vi "Define Mask.vi"(8 "error in (no error)":errorcluster, 11 "FPGA Image":T3(plugin-control)=refnum) -> (0 "error out":errorcluster)   [LabVIEW 2013]
doc: "GUI for selecting a part type and starting a batch process\nPart types list is passed in from caller.\nReturns when Start or Cancel is pressed."
uses:
  Sectors/Number of Wing Sector.ctl
  Mask ROI FG Enum.ctl
  Mask ROI Cluster.ctl
  Common/File IO/INI/Read write mode.ctl
  Message Passing/MsgQ Loops enum.ctl
  System Status/Status FG Enum.ctl
  Common/State Machines/State Machine Lib.lvlib
  Common/GUI/GUI.lvlib
  <vilib>/vision/NI_Vision_Development_Module.lvlib
  Image Processing.lvlib
  Message Passing/Main MsgQ.lvlib
panel:
  in  "Calculate BG":bool
  in  "Load Current Mask":bool
  out "Right ROI":T1 {"Contours"."Type" items=["No Selection", "Point", "Line", "Rectangle", "Oval", "Polygon", "Freehand Region", "Annulus", "Unused2", "Unused3", "Broken Line", "Freehand Line", "Rotated Rectangle"]}
  out "Left ROI":T1 {"Contours"."Type" items=["No Selection", "Point", "Line", "Rectangle", "Oval", "Polygon", "Freehand Region", "Annulus", "Unused2", "Unused3", "Broken Line", "Freehand Line", "Rotated Rectangle"]}
  out "[Avg BG]":dbl[](array[numeric])
  in  "NumWingSectors":T2=1 items=["1"=1, "2"=2, "4"=4, "8"=8, "16"=16]
  out "State":string
  in  "Exit":bool
  in  "Save Mask":bool
  out "combo mask":T3(plugin-control)
  out "right mask":T3(plugin-control)
  out "right masked image":T3(plugin-control)
  out "right annulus":T4={"Center X"=929, "Center Y"=663, "Inner Radius"=200, "Outer Radius"=405, "Start Angle"=90.0, "End Angle"=180.0} {"End Angle" format="%.2f"; "Start Angle" format="%.2f"; "Center X" scale=0.0..1024.0}
  out "left mask":T3(plugin-control)
  out "left masked image":T3(plugin-control)
  out "left annulus":T4={"Center X"=929, "Center Y"=663, "Inner Radius"=200, "Outer Radius"=405, "Start Angle"=90.0, "End Angle"=180.0} {"End Angle" format="%.2f"; "Start Angle" format="%.2f"; "Center X" scale=0.0..1024.0}
  in  "Accept Threshold":bool
  out "Processed Image":T3(plugin-control)
  in  "Threshold Range":cluster{"Lower value":dbl, "Upper value":dbl}={"Lower value"=106.82432432432432, "Upper value"=255.0} {"Upper value" min=0.0 max=255.0 scale=0.0..255.0; "Lower value" min=0.0 max=255.0 scale=0.0..255.0}
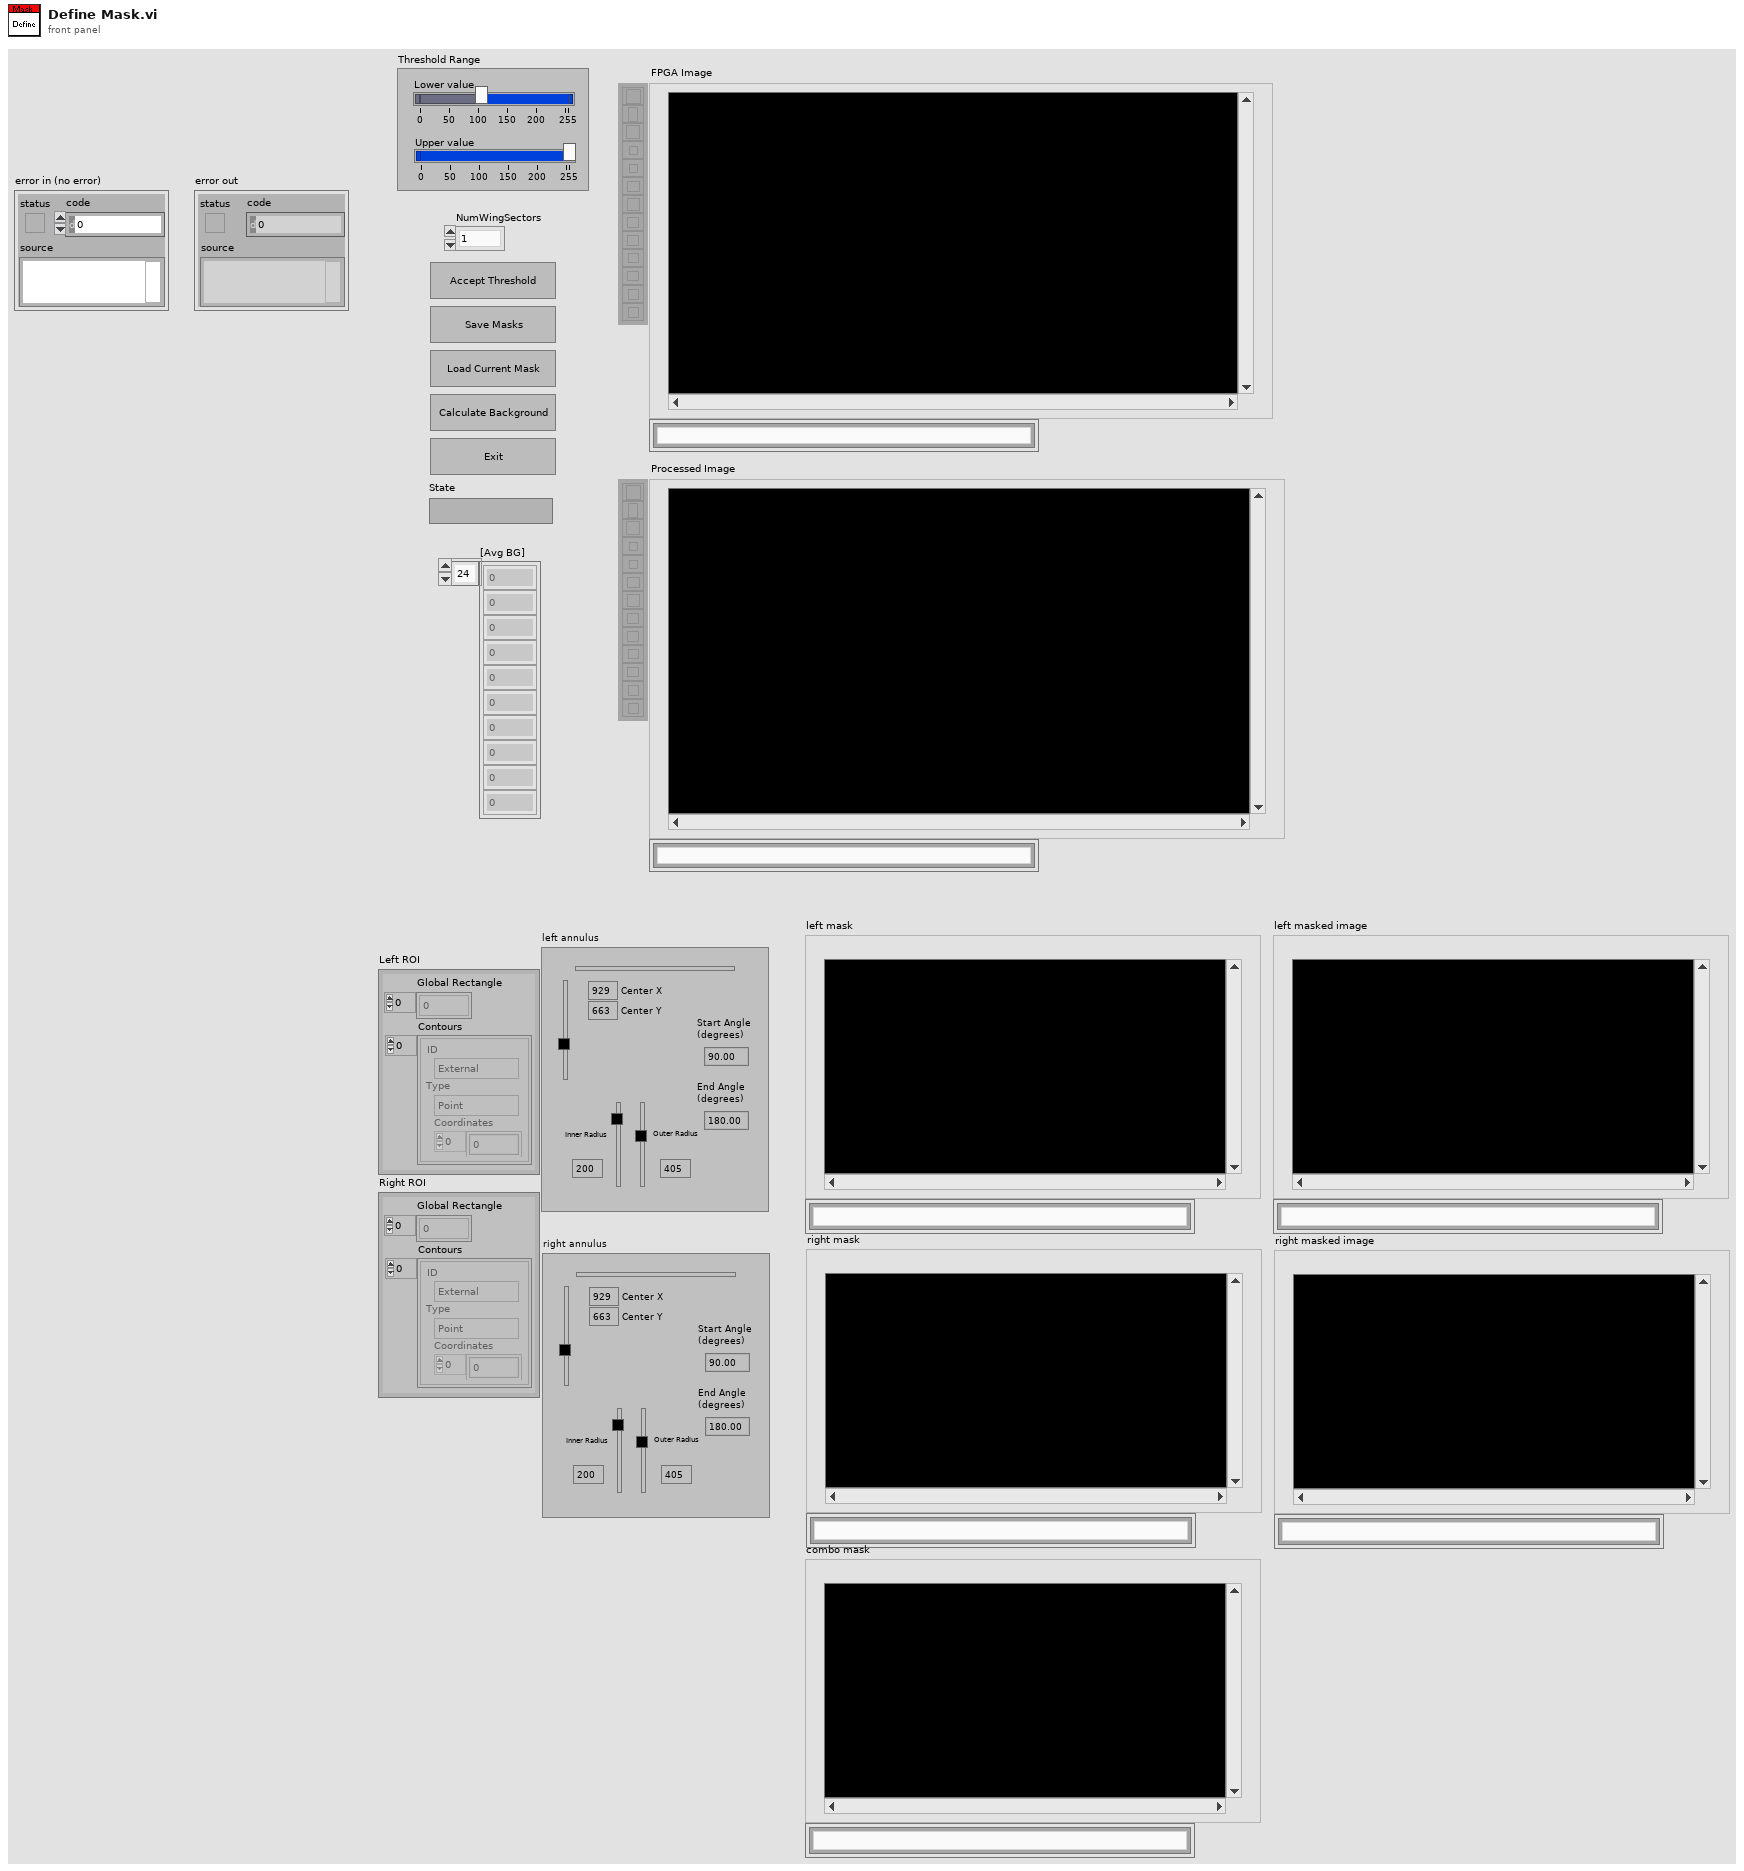
[diagram p1: front panel]
types:
  T1 = typedef "ROI Descriptor" = cluster{"Global Rectangle":i32[], "Contours":cluster{"ID":enum32{"External", "Internal"}, "Type":u32, "Coordinates":i32[]}[]}
  T2 = typedef "Number of Wing Sector.ctl" = u8
  T3 = typedef "IMAQ Image.ctl" = refnum<image>
  T4 = typedef "IMAQ Circle" = cluster{"Center X":i32, "Center Y":i32, "Inner Radius":i32, "Outer Radius":i32, "Start Angle":dbl, "End Angle":dbl}
  T5 = typedef "State Machine Lib.lvlib/STATE cluster.ctl" = cluster{"State":string, "Parameters":variant}
  T6 = typedef "Mask ROI FG Enum.ctl" = enum16{"Read", "Write"}
  T7 = typedef "Main MsgQ.lvlib/MsgQ Loops enum.ctl" = enum16{"User Interface", "Image Acq"}
  T8 = typedef "Read write mode.ctl" = enum16{"Read", "Write"}
  T9 = typedef "Mask ROI Cluster.ctl" = cluster{"left annulus":T4, "right annulus":T4, "Threshold Range":cluster{"Lower value":dbl, "Upper value":dbl}, "[Avg BG]":u8[], "Number of Sectors":u8, "Left ROI":T1, "Right ROI":T1, "Left Start Angle Duty Cycle":fxp<+,8,0>, "Left End Angle Duty Cycle":fxp<+,8,0>, "Right End Angle Duty Cycle":fxp<+,8,0>, "Right Start Angle Duty Cycle":fxp<+,8,0>, "[Sector ROIs]":T1[]}
  T10 = typedef "Status FG Enum.ctl" = enum16{"Reset", "Read", "Write"}
  T11 = typedef "Sector Parameter Cluster.ctl" = cluster{"Start Angle":fxp<+/-,17,2>, "End Angle":fxp<+/-,17,2>, "Inner Radius":u16, "Outter Radius":u16, "Hinge X":u16, "Hinge Y":u16, "NumWingSectors":u8}
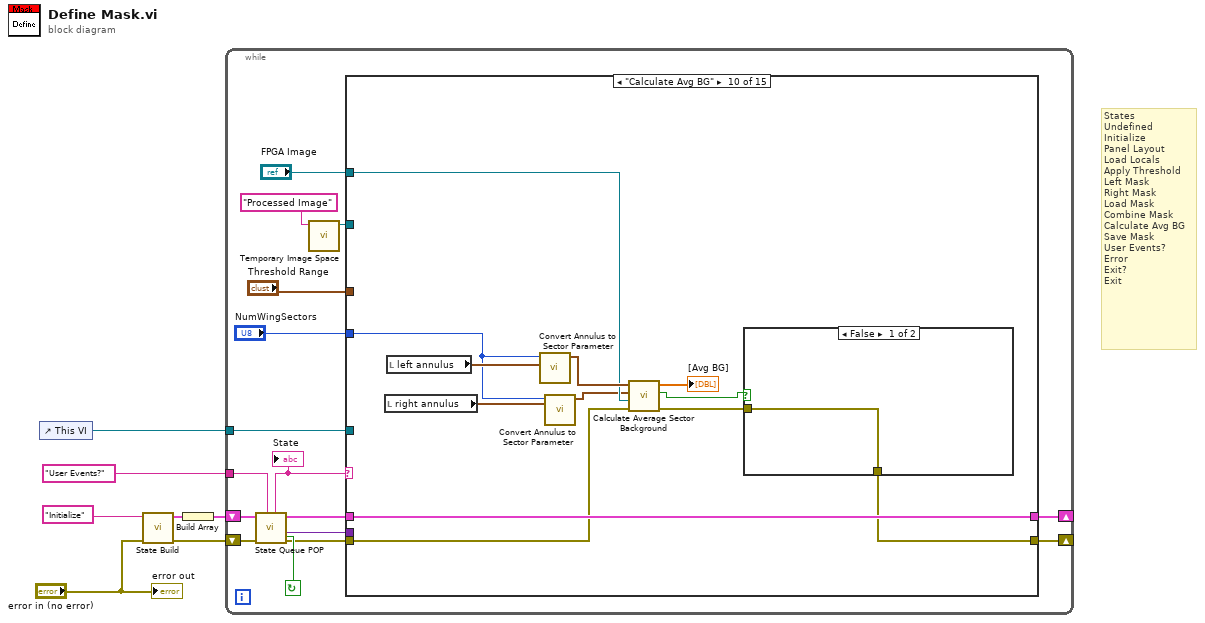
[diagram p0: block diagram]
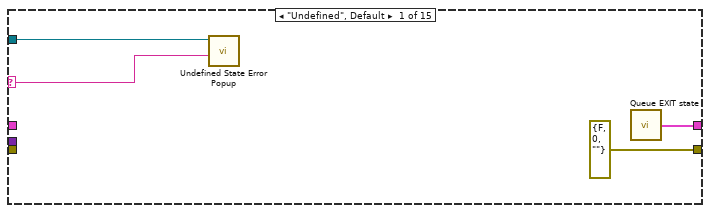
[diagram p2: hidden frame]
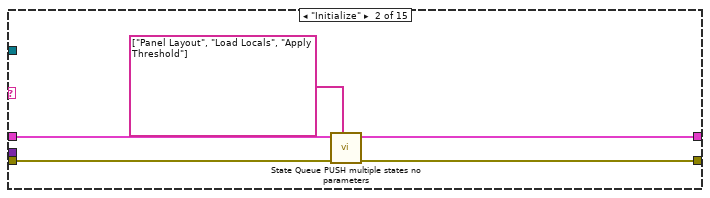
[diagram p3: hidden frame]
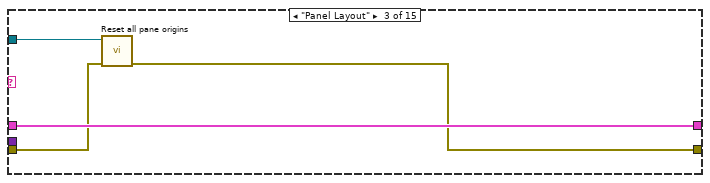
[diagram p4: hidden frame]
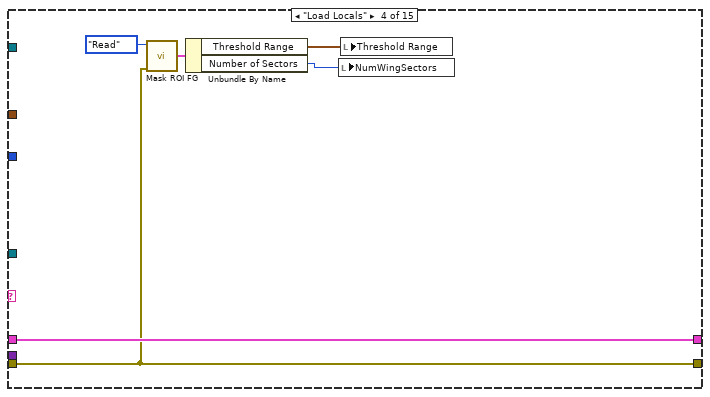
[diagram p5: hidden frame]
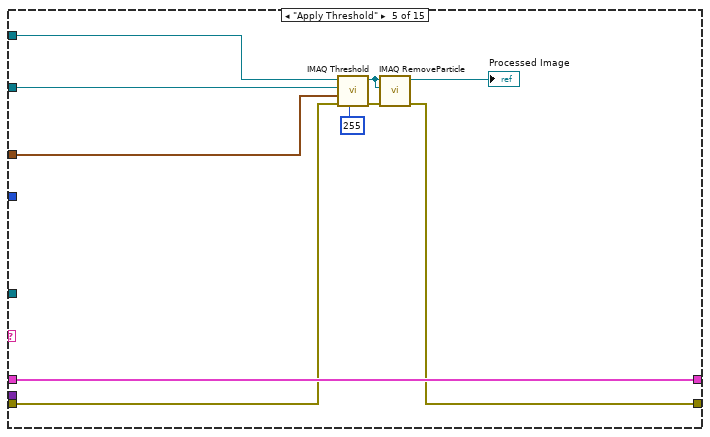
[diagram p6: hidden frame]
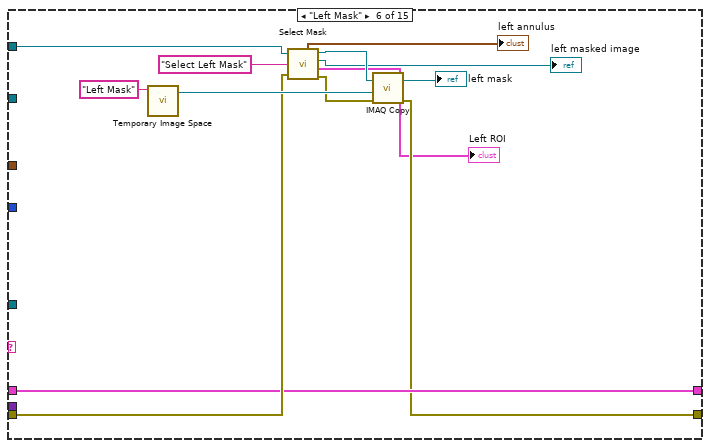
[diagram p7: hidden frame]
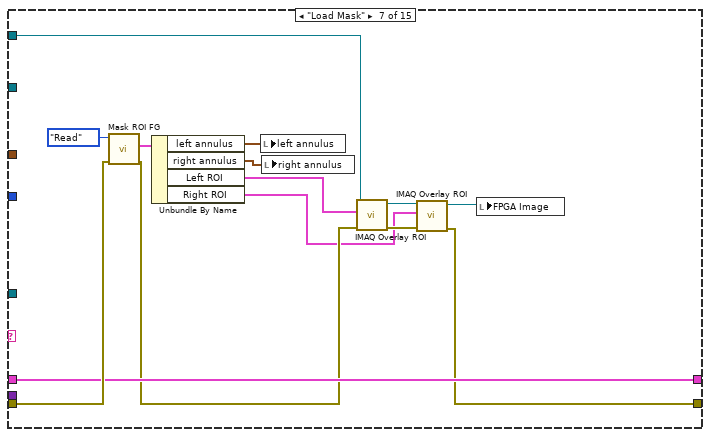
[diagram p8: hidden frame]
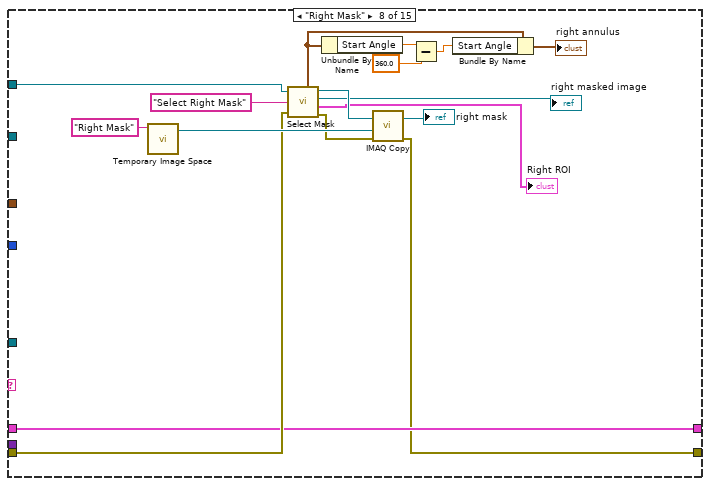
[diagram p9: hidden frame]
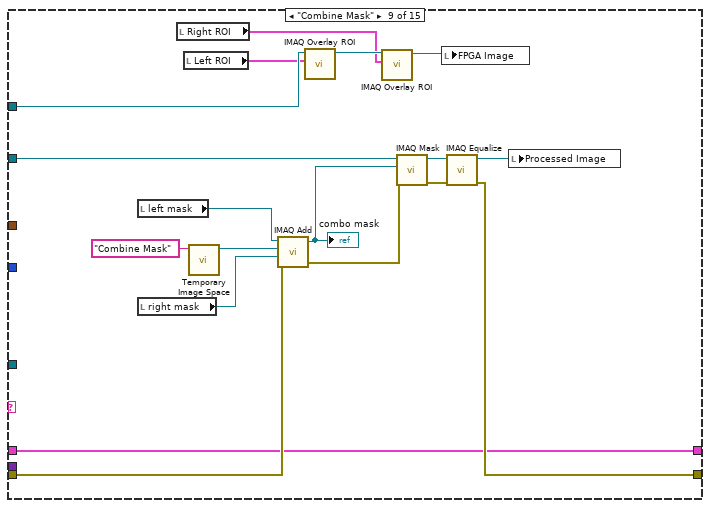
[diagram p10: hidden frame]
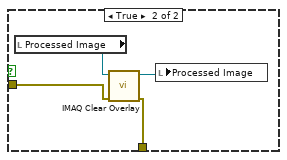
[diagram p11: hidden frame]
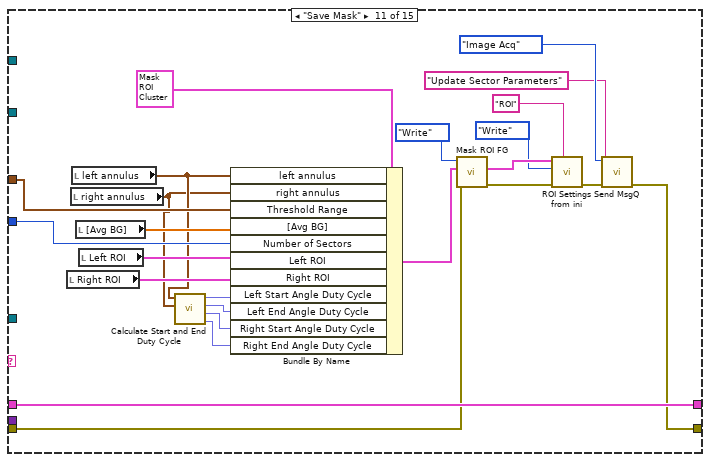
[diagram p12: hidden frame]
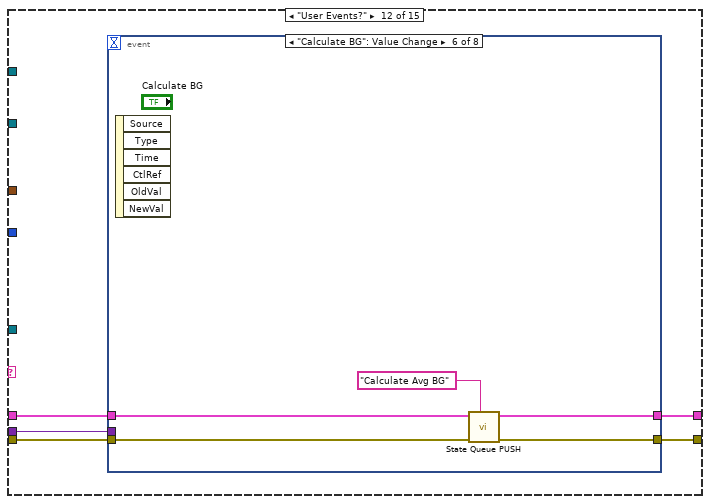
[diagram p13: hidden frame]
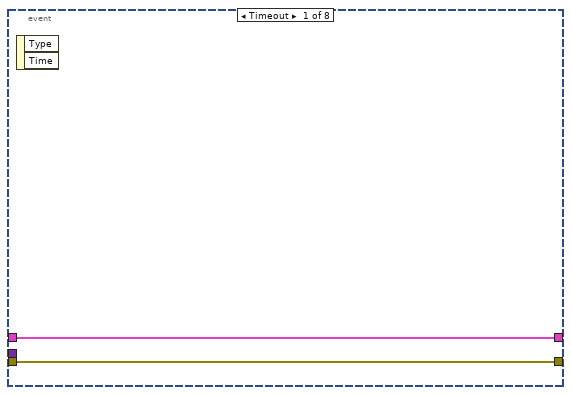
[diagram p14: hidden frame]
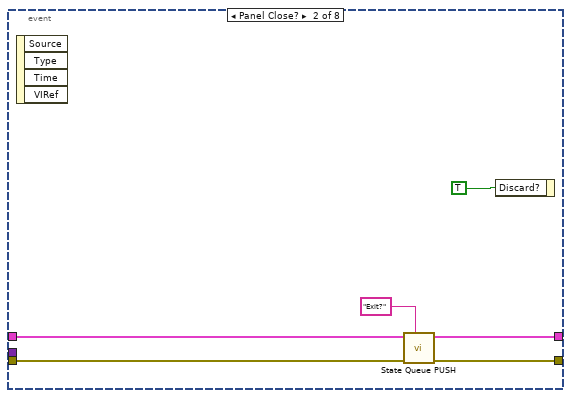
[diagram p15: hidden frame]
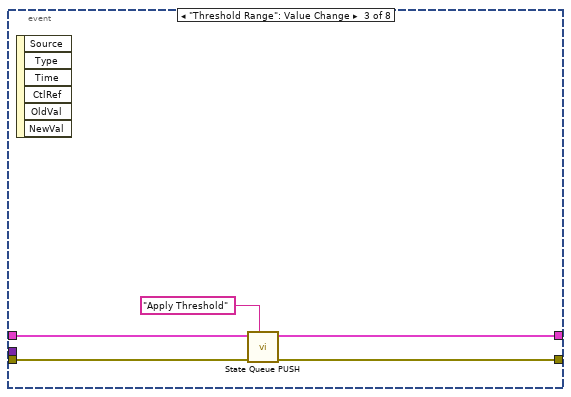
[diagram p16: hidden frame]
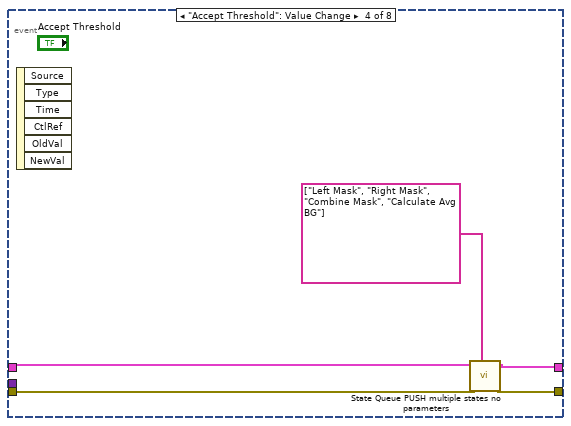
[diagram p17: hidden frame]
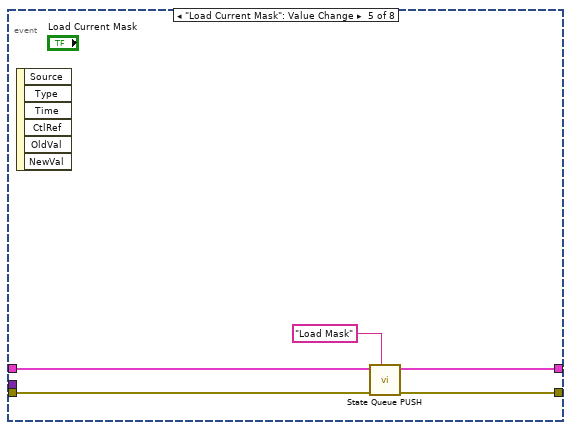
[diagram p18: hidden frame]
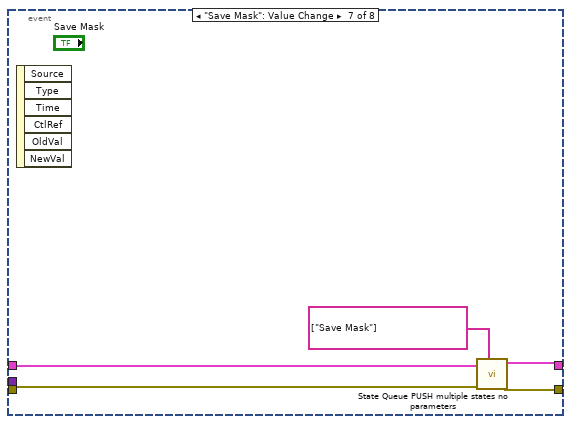
[diagram p19: hidden frame]
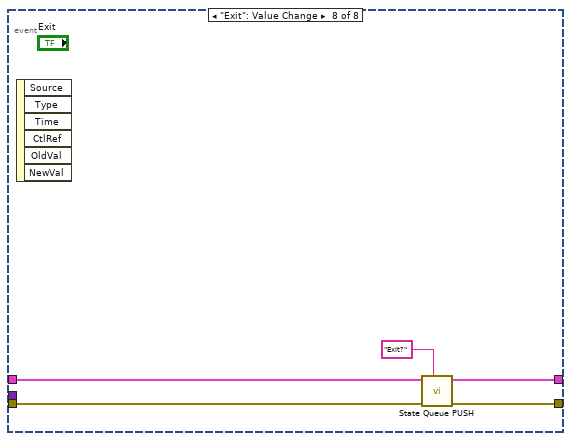
[diagram p20: hidden frame]
diagram:
  # "States\nUndefined\nInitialize\nPanel Layout\nLoad Locals\nApply Threshold\nLeft Mask\nRight Mask\nLoad Mask\nCombine Mask\nCalculate Avg BG\nSave Mask\nUser Events?\nError\nExit?\nExit"
  n1 = control-ref of="This VI"() -> (w6:refnum<vi>)
  n2 = call "State Build.vi"("error in (no error)"="error in (no error)", "State"="Initialize") -> ("error out"=w3:errorcluster, "State Out"=w4:T5)  [unwired: 8 in]
  n3 = Build Array(w4) -> (w5:T5[])
  n4 = while {
    shift-right: [w14] -> _
    shift-left: w3 -> [w22]
    shift-right: [w13] -> _
    shift-left: w5 -> [w20]
    tunnel: "User Events?" ("Default state") -> [w21]
    tunnel: w6 -> [w16]
    stop <- w23 continue-if-true
    n5 = call "State Queue POP.vi"("Default state"=w21, "error in (no error)"=w22, "State que in"=w20) -> ("error out"=w19:errorcluster, "Parameters"=w15:variant, "State que out"=w18:T5[], "Not Exit?"=w23:bool, "State case out"=w17:string)  [unwired: 4 out]
    "State" <- w17
    n6 = call "Temporary Image Space.vi"("Image Name"="Processed Image") -> ("Image Out"=w10:T3)  [unwired: 10 in]
    n7 = case shown="\"Calculate Avg BG\"" w17 {
      selector: w17 -> [w24 _ _ _ _ _ _ _ _ _ _ _ _ _ _]
      tunnel: w19 -> [_ w30 w34 w41 w47 w58 w78 w89 w107 w125 w150 w159 w199 w213 _]
      tunnel: w18 -> [_ w32 w36 w42 w48 w57 w77 w88 w102 w126 w155 w160 _ w207 w215]
      tunnel: w16 -> [w25 _ w35 _ _ _ _ _ _ _ _ _ _ _ _]
      tunnel: w15 -> [_ _ _ _ _ _ _ _ _ _ _ w158 _ _ _]
      tunnel: [errorcluster {"status"=FALSE, "code"=0, "source"=""} ("error out") w31 w33 w41 w46 w56 w68 w87 w103 w116 w140 w157 errorcluster {"status"=FALSE, "code"=0, "source"=""} ("error out") w213 errorcluster {"status"=FALSE, "code"=0, "source"=""} ("error out")] -> w14
      tunnel: [w27 w28 w36 w42 w48 w57 w77 w88 w102 w126 w155 w156 w204 w206 w215] -> w13
      tunnel: "Threshold Range" -> [_ _ _ _ w45 _ _ _ _ _ w152 _ _ _ _]
      tunnel: "FPGA Image" -> [_ _ _ _ w44 w59 w71 w90 w101 w122 _ _ _ _ _]
      tunnel: w10 -> [_ _ _ _ w43 _ _ _ w106 _ _ _ _ _ _]
      tunnel: "NumWingSectors" -> [_ _ _ _ _ _ _ _ _ w120 w148 _ _ _ _]
      frame "Undefined", Default {
        n8 = call "Undefined State Error Popup.vi"("String"=w24, "This VI (Caller if unwired)"=w25) -> ()  [unwired: 10 out]
        n9 = call "Queue EXIT state.vi"() -> ("Exit State Q"=w27:T5[])  [unwired: 1 in]
      }
      frame "Initialize" {
        n10 = call "State Queue PUSH multiple states no parameters.vi"("States to queue"=string[] ["Panel Layout", "Load Locals", "Apply Threshold"], "error in (no error)"=w30, "State que in"=w32) -> ("error out"=w31:errorcluster, "State que out"=w28:T5[])  [unwired: 1 in, 6 out]
      }
      frame "Panel Layout" {
        n11 = call "Reset all pane origins.vi"("error in (no error"=w34, "Vi Ref In"=w35) -> ("error out"=w33:errorcluster)  [unwired: 9 out]
      }
      frame "Load Locals" {
        n12 = call "Mask ROI FG.vi"("error in (no error)"=w41, "Operation"=Mask_ROI_FG_Enum."Read") -> ("Mask ROI Out"=w39:T9)  [unwired: 8 in, 1 out]
        n13 = Unbundle By Name(w39) -> ("Threshold Range"=w38:cluster{"Lower value":dbl, "Upper value":dbl}, "Number of Sectors"=w37:u8)
        n14 = local write "NumWingSectors"(w37) -> ()
        n15 = local write "Threshold Range"(w38) -> ()
      }
      frame "Apply Threshold" {
        n16 = call "IMAQ Threshold"("Replace Value"=u8 255, "error in (no error)"=w47, "Range"=w45, "Image Dst"=w43, "Image Src"=w44) -> ("error out"=w50:errorcluster, "Image Dst Out"=w52:T3)  [unwired: 1 in, 4 out]
        n17 = call "IMAQ RemoveParticle"("error in (no error)"=w50, "Image Dst"=w52, "Image Src"=w52) -> ("error out"=w46:errorcluster, "Image Dst Out"=→"Processed Image":T3)  [unwired: 4 in, 3 out]
      }
      frame "Left Mask" {
        n18 = call "Temporary Image Space.vi"("Image Name"="Left Mask") -> ("Image Out"=w60:T3)  [unwired: 10 in]
        n19 = call "Select Mask.vi"("error in"=w58, "Prompt"="Select Left Mask", "Read \nImage"=w59) -> ("error out"=w55:errorcluster, "ROI Descriptor Out"=→"Left ROI":T1, "Masked \nImage"=→"left masked image":T3, "Annulus"=→"left annulus":T4, "mask"=w63:T3)  [unwired: 1 out]
        n20 = call "IMAQ Copy"("error in (no error)"=w55, "Image Dst"=w60, "Image Src"=w63) -> ("error out"=w56:errorcluster, "Image Dst Out"=→"left mask":T3)  [unwired: 3 in]
      }
      frame "Load Mask" {
        n21 = call "Mask ROI FG.vi"("error in (no error)"=w78, "Operation"=Mask_ROI_FG_Enum."Read") -> ("error out"=w69:errorcluster, "Mask ROI Out"=w76:T9)  [unwired: 8 in]
        n22 = Unbundle By Name(w76) -> ("left annulus"=w75:T4, "right annulus"=w74:T4, "Left ROI"=w67:T1, "Right ROI"=w66:T1)
        n23 = local write "left annulus"(w75) -> ()
        n24 = local write "right annulus"(w74) -> ()
        n25 = call "IMAQ Overlay ROI"("error in (no error)"=w69, "ROI Descriptor"=w67, "Image"=w71) -> ("error out"=w70:errorcluster, "Image Out"=w73:T3)  [unwired: 7 in]
        n26 = call "IMAQ Overlay ROI"("error in (no error)"=w70, "ROI Descriptor"=w66, "Image"=w73) -> ("error out"=w68:errorcluster, "Image Out"=w72:T3)  [unwired: 7 in]
        n27 = local write "FPGA Image"(w72) -> ()
      }
      frame "Right Mask" {
        n28 = call "Temporary Image Space.vi"("Image Name"="Right Mask") -> ("Image Out"=w91:T3)  [unwired: 10 in]
        n29 = call "Select Mask.vi"("error in"=w89, "Prompt"="Select Right Mask", "Read \nImage"=w90) -> ("error out"=w86:errorcluster, "ROI Descriptor Out"=→"Right ROI":T1, "Masked \nImage"=→"right masked image":T3, "Annulus"=w80:T4, "mask"=w94:T3)  [unwired: 1 out]
        n30 = Unbundle By Name(w80) -> ("Start Angle"=w85:dbl)
        n31 = call "IMAQ Copy"("error in (no error)"=w86, "Image Dst"=w91, "Image Src"=w94) -> ("error out"=w87:errorcluster, "Image Dst Out"=→"right mask":T3)  [unwired: 3 in]
        n32 = Subtract(x=w85, y=360.0) -> (x-y=w83:dbl)
        n33 = Bundle By Name(cluster=w80, "Start Angle"=w83) -> (→"right annulus":T4)
      }
      frame "Combine Mask" {
        n34 = local read "left mask"() -> (w109:T3)
        n35 = local read "right mask"() -> (w108:T3)
        n36 = local read "Right ROI"() -> (w98:T1)
        n37 = local read "Left ROI"() -> (w100:T1)
        n38 = call "Temporary Image Space.vi"("Image Name"="Combine Mask") -> ("Image Out"=w111:T3)  [unwired: 10 in]
        n39 = call "IMAQ Add"("Image Src A"=w109, "Image Dst"=w111, "Image Src B"=w108, "error in (no error)"=w107) -> ("Image Dst Out"=w112:T3, "error out"=w104:errorcluster)  [unwired: 3 in]
        "combo mask" <- w112
        n40 = call "IMAQ Overlay ROI"("ROI Descriptor"=w100, "Image"=w101) -> ("Image Out"=w99:T3)  [unwired: 8 in, 1 out]
        n41 = call "IMAQ Overlay ROI"("ROI Descriptor"=w98, "Image"=w99) -> ("Image Out"=w97:T3)  [unwired: 8 in, 1 out]
        n42 = call "IMAQ Mask"("error in (no error)"=w104, "Image Mask"=w112, "Image Src"=w106) -> ("error out"=w113:errorcluster, "Image Dst Out"=w114:T3)  [unwired: 1 in, 1 out]
        n43 = local write "FPGA Image"(w97) -> ()
        n44 = call "IMAQ Equalize"("error in (no error)"=w113, "Image Src"=w114) -> ("error out"=w103:errorcluster, "Image Dst Out"=w105:T3)  [unwired: 4 in, 4 out]
        n45 = local write "Processed Image"(w105) -> ()
      }
      frame "Calculate Avg BG" {
        n46 = local read "right annulus"() -> (w119:T4)
        n47 = local read "left annulus"() -> (w124:T4)
        n48 = call "Convert Annulus to Sector Parameter.vi"("Annulus"=w124, "NumWingSectors"=w120) -> ("Sector Parameter"=w123:T11)  [unwired: 9 in]
        n49 = call "Convert Annulus to Sector Parameter.vi"("Annulus"=w119, "NumWingSectors"=w120) -> ("Sector Parameter"=w118:T11)  [unwired: 9 in]
        n50 = call "Calculate Average Sector Background.vi"("error in (no error)"=w125, "Image"=w122, "Right Sector Parameters"=w118, "Left Sector Parameters"=w123) -> ("error out"=w117:errorcluster, "Canceled?"=w115:bool, "[Avg BG]"=→"[Avg BG]":dbl[])  [unwired: 5 in]
        n51 = case shown="False" w115 {
          tunnel: w117 -> [w127 w130]
          tunnel: [w127 w129] -> w116
          frame False {
          }
          frame True {
            n52 = local read "Processed Image"() -> (w131:T3)
            n53 = call "IMAQ Clear Overlay"("error in (no error)"=w130, "Image"=w131) -> ("error out"=w129:errorcluster, "Image Out"=w128:T3)  [unwired: 8 in]
            n54 = local write "Processed Image"(w128) -> ()
          }
        }
      }
      frame "Save Mask" {
        n55 = local read "Right ROI"() -> (w138:T1)
        n56 = local read "right annulus"() -> (w136:T4)
        n57 = local read "left annulus"() -> (w137:T4)
        n58 = local read "[Avg BG]"() -> (w149:dbl[])
        n59 = local read "Left ROI"() -> (w139:T1)
        n60 = call "Calculate Start and End Duty Cycle.vi"("right annulus"=w136, "left annulus"=w137) -> ("Right End Angle Duty Cycle"=w132:fxp<+,8,0>, "Right Start Angle Duty Cycle"=w133:fxp<+,8,0>, "Left End Angle Duty Cycle"=w134:fxp<+,8,0>, "Left Start Angle Duty Cycle"=w135:fxp<+,8,0>)  [unwired: 6 in]
        n61 = Bundle By Name(cluster=T9 {"left annulus"={"Center X"=929, "Center Y"=663, "Inner Radius"=200, "Outer Radius"=405, "Start Angle"=90.0, "End Angle"=180.0}, "right annulus"={"Center X"=929, "Center Y"=663, "Inner Radius"=200, "Outer Radius"=405, "Start Angle"=90.0, "End Angle"=180.0}, "Threshold Range"={"Lower value"=106.82432432432432, "Upper value"=255.0}, "[Avg BG]"=[], "Number of Sectors"=0, "Left ROI"={"Global Rectangle"=[], "Contours"=[]}, "Right ROI"={"Global Rectangle"=[], "Contours"=[]}, "Left Start Angle Duty Cycle"=0.0, "Left End Angle Duty Cycle"=0.0, "Right End Angle Duty Cycle"=0.0, "Right Start Angle Duty Cycle"=0.0, "[Sector ROIs]"=[]} ("Mask ROI In"), "left annulus"=w137, "right annulus"=w136, "Threshold Range"=w152, "[Avg BG]"=w149, "Number of Sectors"=w148, "Left ROI"=w139, "Right ROI"=w138, "Left Start Angle Duty Cycle"=w135, "Left End Angle Duty Cycle"=w134, "Right Start Angle Duty Cycle"=w133, "Right End Angle Duty Cycle"=w132) -> (w151:T9)
        n62 = call "Mask ROI FG.vi"("error in (no error)"=w150, "Mask ROI In"=w151, "Operation"=Mask_ROI_FG_Enum."Write") -> ("error out"=w145:errorcluster, "Mask ROI Out"=w147:T9)  [unwired: 7 in]
        n63 = call "ROI Settings from ini.vi"("Section"="ROI", "error in (no error)"=w145, "Operation"=Read_write_mode."Write", "Mask ROI In"=w147) -> ("error out"=w141:errorcluster)  [unwired: 5 in, 2 out]
        n64 = call "Send MsgQ.vi"("error in (no error)"=w141, "Message String"="Update Sector Parameters", "Send to MsgQ"=MsgQ_Loops_enum."Image Acq") -> ("error out"=w140:errorcluster)  [unwired: 8 in]
      }
      frame "User Events?" {
        n65 = event shown="[5] \"Calculate BG\": Value Change" {
          selector: _ -> [_ _ _ _ _ _ _ _]
          dyn-events: _ -> [_ _ _ _ _ _ _ _]
          timeout: _ -> [_ _ _ _ _ _ _ _]
          tunnel: w160 -> [w161 w167 w173 w176 w182 w187 w192 w195]
          tunnel: w159 -> [w162 w166 w172 w174 w179 w184 w189 w196]
          tunnel: w158 -> [_ _ _ _ _ _ _ _]
          tunnel: [w162 w164 w170 w177 w180 w185 w190 w197] -> w157
          tunnel: [w161 w165 w171 w178 w181 w186 w191 w198] -> w156
          event Timeout {
            n66 = event-data() -> ()  [unwired: 3 out]
          }
          event Panel Close? {
            n67 = event-data() -> ()  [unwired: 5 out]
            n68 = call "State Queue PUSH.vi"("State case"="Exit?", "error in (no error)"=w166, "State que in"=w167) -> ("error out"=w164:errorcluster, "State que out"=w165:T5[])  [unwired: 2 in, 5 out]
            n69 = event-data("Discard?"=TRUE) -> ()  [unwired: 1 in, 1 out]
          }
          event "Threshold Range": Value Change {
            n70 = event-data() -> ()  [unwired: 7 out]
            n71 = call "State Queue PUSH.vi"("State case"="Apply Threshold", "error in (no error)"=w172, "State que in"=w173) -> ("error out"=w170:errorcluster, "State que out"=w171:T5[])  [unwired: 2 in, 5 out]
          }
          event "Accept Threshold": Value Change {
            n72 = event-data() -> ()  [unwired: 7 out]
            n73 = call "State Queue PUSH multiple states no parameters.vi"("States to queue"=string[] ["Left Mask", "Right Mask", "Combine Mask", "Calculate Avg BG"], "error in (no error)"=w174, "State que in"=w176) -> ("error out"=w177:errorcluster, "State que out"=w178:T5[])  [unwired: 7 in]
          }
          event "Load Current Mask": Value Change {
            n74 = event-data() -> ()  [unwired: 7 out]
            n75 = call "State Queue PUSH.vi"("State case"="Load Mask", "error in (no error)"=w179, "State que in"=w182) -> ("error out"=w180:errorcluster, "State que out"=w181:T5[])  [unwired: 2 in, 5 out]
          }
          event "Calculate BG": Value Change {
            n76 = event-data() -> ()  [unwired: 7 out]
            n77 = call "State Queue PUSH.vi"("State case"="Calculate Avg BG", "error in (no error)"=w184, "State que in"=w187) -> ("error out"=w185:errorcluster, "State que out"=w186:T5[])  [unwired: 2 in, 5 out]
          }
          event "Save Mask": Value Change {
            n78 = event-data() -> ()  [unwired: 7 out]
            n79 = call "State Queue PUSH multiple states no parameters.vi"("States to queue"=string[] ["Save Mask"], "error in (no error)"=w189, "State que in"=w192) -> ("error out"=w190:errorcluster, "State que out"=w191:T5[])  [unwired: 7 in]
          }
          event "Exit": Value Change {
            n80 = event-data() -> ()  [unwired: 7 out]
            n81 = call "State Queue PUSH.vi"("State case"="Exit?", "error in (no error)"=w196, "State que in"=w195) -> ("error out"=w197:errorcluster, "State que out"=w198:T5[])  [unwired: 7 in]
          }
        }
      }
      frame "Error" {
        # "DEFAULT IS \nTO CLEAR ERROR\nAND EXIT"
        n82 = Unbundle By Name(w199) -> ("source"=w202:string)
        n83 = Concatenate Strings("Error: " ("string"), w202) -> (w201:string)
        n84 = call "Status FG.vi"("Status In"=w201, "Operation"=Status_FG_Enum."Write") -> ()  [unwired: 8 in, 2 out]
        n85 = call <vilib>:"Clear Errors.vi"("error in (no error)"=w199) -> ()  [unwired: 7 out]
        n86 = call "Queue EXIT state.vi"() -> ("Exit State Q"=w204:T5[])  [unwired: 1 in]
      }
      frame "Exit?" {
        n87 = Two Button Dialog(message="Exit?", 1:"No" ("F button name (\"Cancel\")"), 2:"Yes" ("T button name (\"OK\")")) -> (T button?=w209:bool)
        n88 = call "Queue EXIT state.vi"() -> ("Exit State Q"=w208:T5[])  [unwired: 1 in]
        n89 = Select(t=w208, s=w209, f=w207) -> (s? t:f=w206:T5[])
      }
      frame "Exit" {
      }
    }
  }
  "error out" <- "error in (no error)"
